vi "tdms_read_by1.vi"(4 "error in":errorcluster, 5 "filter":bool, 6 "Array 3":string[](array[string])=["phase_a", "phase_b", "phase_c"], 7 "datalog path":path) -> (0 "error out":errorcluster, 1 "Array 2":cluster{"f0":dbl, "df":dbl, "magnitude":dbl[]}[](array[cluster]), 2 "Array":waveform(i16)[](array[waveform]), 3 "file path out":path)   [LabVIEW 2010]
uses:
  <vilib>/express/express analysis/Spectral/XNode/ExpressSpectralMeasurementsBlockNode.xnode
  math/mean12.vi
  <vilib>/express/express analysis/Spectral/Block/exnSpectralBlock spectral measurements peak poly.vi
  <vilib>/express/express analysis/Spectral/Block/exnSpectralBlock spectral measurements peak WFM.vi
panel:
  out "mean_dy_std":dbl[][](array[numeric])
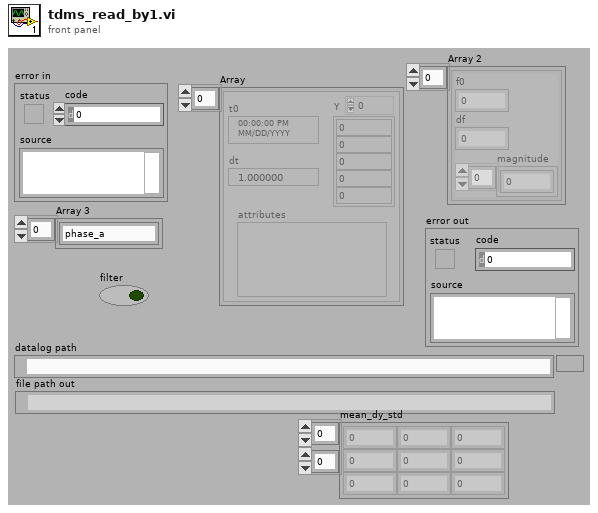
[diagram p1: front panel]
types:
  T1 = enum16{"open", "open or create", "create or replace", "create", "open (read-only)"}
  T2 = cluster{"averaging mode":u16, "weighting mode":u16, "number of averages":u32}
  T3 = cluster{"dB On (F)":bool, "unwrap phase (F)":bool, "convert to degree (F)":bool}
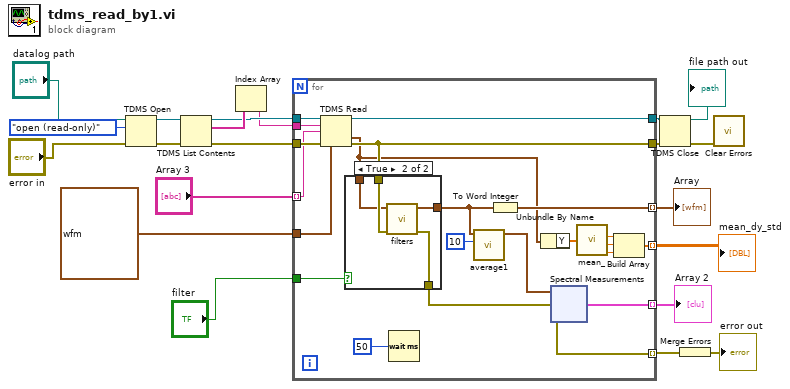
[diagram p0: block diagram]
diagram:
  n1 = TDMS Open(8:"error in", 10:T1."open (read-only)" ("operation (0:open)"), 11:"datalog path") -> (0:w9:errorcluster, 3:w10:refnum<k34>)  [unwired: 3 in]
  n2 = TDMS List Contents(4:w9, 7:w10) -> (0:w7:errorcluster, 2:w11:string[], 3:w8:refnum<k34>)  [unwired: 1 in, 1 out]
  n3 = Index Array(array=w11) -> (element=w6:string)  [unwired: 1 in]
  n4 = for {
    tunnel: w6 -> [w43]
    tunnel: w7 -> [w42]
    tunnel: w8 -> [w41]
    tunnel: [w40] -> w21
    tunnel: [w36] -> w20
    tunnel: waveform(dbl) {"t0"=timestamp(0 s since 1904-01-01), "dt"=1.0, "Y"=[]} ("data") -> [w39]
    tunnel: "Array 3" -> [w38] mode=indexing
    tunnel: [w27] -> w18 mode=indexing
    tunnel: [w37] -> w17 mode=indexing
    tunnel: "filter" -> [w31]
    tunnel: [w30] -> w4 mode=indexing
    tunnel: [w22] -> w1 mode=indexing
    n5 = TDMS Read(0:w41, 5:w43, 7:w38, 11:w42, 12:w39) -> (4:w40:refnum<k34>, 10:w26:waveform(dbl), 15:w36:errorcluster)  [unwired: 2 in, 3 out]
    n6 = case shown="True" w31 {
      tunnel: w36 -> [w44 w49]
      tunnel: w26 -> [w45 w48]
      tunnel: [w45 w47] -> w33
      tunnel: [w44 w46] -> w32
      frame False {
      }
      frame True {
        n7 = call "filters.vi"("error in (no error)"=w49, "Waveform"=w48) -> ("error out"=w46:errorcluster, "SignalOut"=w47:waveform(dbl))  [unwired: 4 in]
      }
    }
    n8 = Wait (ms)(milliseconds to wait=u32 50) -> ()  [unwired: 1 out]
    n9 = call "average1.vi"("Size"=10, "SignalIn"=w33) -> ("output waveform"=w35:waveform(dbl))  [unwired: 5 in]
    n10 = To Word Integer(number=w33) -> (16bit integer=w27:waveform(i16))
    n11 = Unbundle By Name(w26) -> ("Y"=w28:dbl[])
    n12 = xnode "Spectral Measurements"("Signals"=w35, "error in (no error)"=w32) -> ("FFT - (Peak)"=w37:cluster{"f0":dbl, "df":dbl, "magnitude":dbl[]}, "error out"=w30:errorcluster)  [unwired: 1 out]
    n13 = call-poly "mean_.vi"("Y"=w28) -> ("mean"=w25:dbl, "dY"=w24:dbl, "std"=w23:dbl)  [unwired: 5 in]
    n14 = Build Array(w25, w24, w23) -> (w22:dbl[])
  }
  "Array" <- w18
  "Array 2" <- w17
  "mean_dy_std" <- w1
  n15 = TDMS Close(8:w20, 11:w21) -> (0:w15:errorcluster, 3:→"file path out":path)
  n16 = Merge Errors(w4) -> (→"error out":errorcluster)
  n17 = call <vilib>:"Clear Errors.vi"("error in (no error)"=w15) -> ()  [unwired: 6 in, 1 out]
